vi "Create Publisher.vi"(8 "error in (no error)":errorcluster, 9 "Default Value":dbl, 10 "Name":string, 11 "RTFIFODouble in":refnum<class "CIFTag.lvclass">) -> (0 "error out":errorcluster, 3 "RTFIFODouble out":refnum<class "CIFTag.lvclass">)   [LabVIEW 2021, in "CIFTag.lvclass"]
uses:
  CIFTag.lvclass
  D:/dev/CIF-LVCore/src/CIFUtilities/CIFChannels/CIFChannels.lvclass
  CIFUtilities/CIFChannels/Typedef/Direction.ctl
  CIFUtilities/CIFChannels/Typedef/Disconnect Behavior.ctl
  CIFUtilities/CIFChannels/Typedef/Channel State.ctl
  CIFUtilities/CIFChannels/CIFChannels.lvclass/CIFChannels.ctl
  CIFTag.lvclass/CIFTag.ctl
  CIFUtilities/CIFChannels/Accessors/Write Channel State.vi
  CIFUtilities/CIFChannels/Write Channel Class.vi
  CIFUtilities/CIFChannels/Accessors/Write Direction.vi
  CIFUtilities/CIFChannels/Accessors/Write Disconnect Behavior.vi
  CIFUtilities/CIFChannels/Accessors/Write Name.vi
  CIFUtilities/CIFChannels/Accessors/Write Stored Data.vi
  <vilib>/Utility/LVClass/Get LV Class Name.vi
  CIFUtilities/CIFChannels/CIFChannels.lvclass
  D:/dev/CIF-LVCore/src/Channels/CIFChannel/CIFTag.lvclass
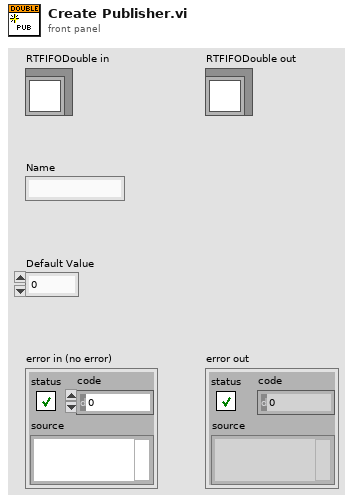
[diagram p1: front panel]
types:
  T1 = typedef "CIFChannels.lvclass/Channel State.ctl" = enum16{"Creating", "Disconnected", "Connecting", "Connected", "Destroying"}
  T2 = cluster{"read mode":enum16{"polling", "blocking"}, "write mode":enum16{"polling", "blocking"}}
  T3 = typedef "CIFChannels.lvclass/Disconnect Behavior.ctl" = enum16{"Default value", "Last value", "Error with default"}
  T4 = typedef "CIFChannels.lvclass/Direction.ctl" = enum16{"Publisher", "Subscriber"}
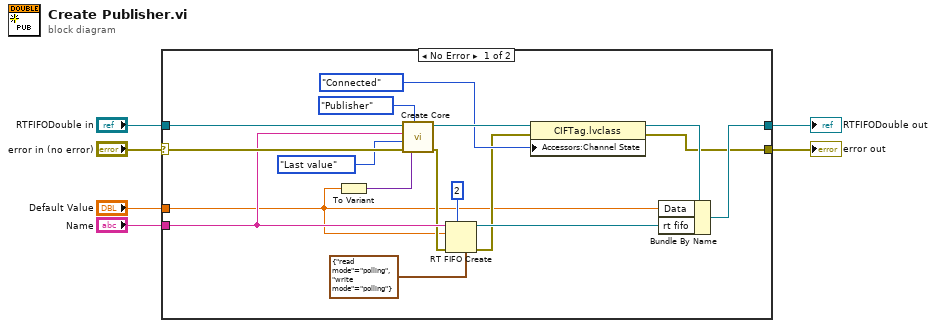
[diagram p0: block diagram]
diagram:
  n1 = case shown="No Error" "error in (no error)" {
    selector: "error in (no error)" -> [w21 w25]
    tunnel: [w8 w25] -> w5
    tunnel: [w13 w24] -> w3
    tunnel: "RTFIFODouble in" -> [w23 w24]
    tunnel: "Name" -> [w18 _]
    tunnel: "Default Value" -> [w7 _]
    frame No Error {
      n2 = To Variant(anything=w7) -> (Variant=w19:variant)
      n3 = call "Create Core.vi"("Stored Data"=w19, "Direction"=Direction."Publisher", "error in (no error)"=w21, "Disconnect Behavior"=Disconnect_Behavior."Last value", "Name"=w18, "CIFChannels in"=w23) -> ("error out"=w10:errorcluster, "CIFChannels in"=w14:refnum<class "CIFTag.lvclass">)  [unwired: 4 in]
      n4 = RT FIFO Create(0:w18, 1:w7, 3:w10, 4:u32 2 ("size (10)"), 7:T2 {"read mode"=enum."polling", "write mode"=enum."polling"} ("r/w modes (polling,polling)")) -> (8:w15:refnum<k33>, 11:w9:errorcluster)  [unwired: 3 in, 1 out]
      n5 = property class="CIFTag.lvclass"(reference=w14, error in=w9, "Accessors:Channel State"=Channel_State."Connected" ("Channel State")) -> (reference out=w12:refnum<class "CIFTag.lvclass">, error out=w8:errorcluster)
      n6 = Bundle By Name(cluster=w12, "Data"=w7, "rt fifo"=w15) -> (w13:refnum<class "CIFTag.lvclass">)
    }
    frame Error {
    }
  }
  "error out" <- w5
  "RTFIFODouble out" <- w3
